vi "SwerveBegin.vi"() -> ()   [LabVIEW 2019]
uses:
  <vilib>/Rock Robotics/WPI/ThirdParty/Phoenix-LabVIEW/Motor Controller/Controls/CTRE_Phoenix_MotorControl_NeutralMode.ctl
panel:
  in  "PIDF":cluster{"P":dbl, "I":dbl, "D":dbl, "F":dbl}={"P"=0.1, "I"=0.0, "D"=0.0, "F"=0.0} {"P" format="%#_13g"}
  in  "Error In":errorcluster
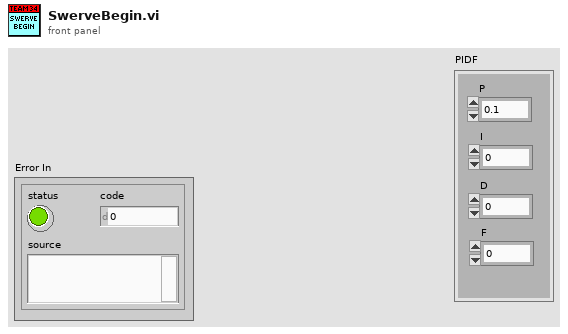
[diagram p1: front panel]
types:
  T1 = typedef "CTRE_Phoenix_MotorControl_NeutralMode.ctl" = enum8{"EEPROMSetting", "Override to Coast", "Override to Brake"}
  T2 = typedef "WPI_MotorControlDeviceRef.ctl" = cluster{"DeviceStatus":errorcluster, "Type":T3, "PWM":cluster{"PWM Channel":T4, "DeadBand":T5}, "CAN":cluster{"Device Number":u8, "SetOutput VI Ref":variant, "GetOutput VI Ref":variant, "Enable VI Ref":variant, "Disable VI Ref":variant, "Data":variant}, "Invert":bool, "DIO PWM":cluster{"PWM \"Enable\" Channel":T4, "DIOChannel":T6, "PWM Rate":dbl}}
  T3 = typedef "WPI_MotorControlType.ctl" = enum16{"PWM", "CAN", "DIO PWM"}
  T4 = typedef "FPGA_DIOPWMChannel.ctl" = enum8{"PWM 0", "PWM 1", "PWM 2", "PWM 3", "PWM 4", "PWM 5", "PWM 6", "PWM 7", "PWM 8", "PWM 9", "PWM MXP 0", "PWM MXP 1", "PWM MXP 2", "PWM MXP 3", "PWM MXP 4", "PWM MXP 5", "PWM MXP 6", "PWM MXP 7", "PWM MXP 8", "PWM MXP 9", "Invalid"}
  T5 = typedef "WPI_PWMDeadband.ctl" = cluster{"Name":string, "maxPositivePwm":i32, "minPositivePwm":i32, "centerPwm":i32, "maxNegativePwm":i32, "minNegativePwm":i32, "angularRange":u16}
  T6 = typedef "FPGA_DIOChannel.ctl" = enum8{"DIO 0", "DIO 1", "DIO 2", "DIO 3", "DIO 4", "DIO 5", "DIO 6", "DIO 7", "DIO 8", "DIO 9", "DIO MXP 0", "DIO MXP 1", "DIO MXP 2", "DIO MXP 3", "DIO MXP 4", "DIO MXP 5", "DIO MXP 6", "DIO MXP 7", "DIO MXP 8", "DIO MXP 9", "DIO MXP 10", "DIO MXP 11", "DIO MXP 12", "DIO MXP 13", "DIO MXP 14", "DIO MXP 15", "SPI Port CS1", "SPI Port CS2", "SPI Port CS3", "SPI Port MISO", "SPI Port MOSI", "Invalid"}
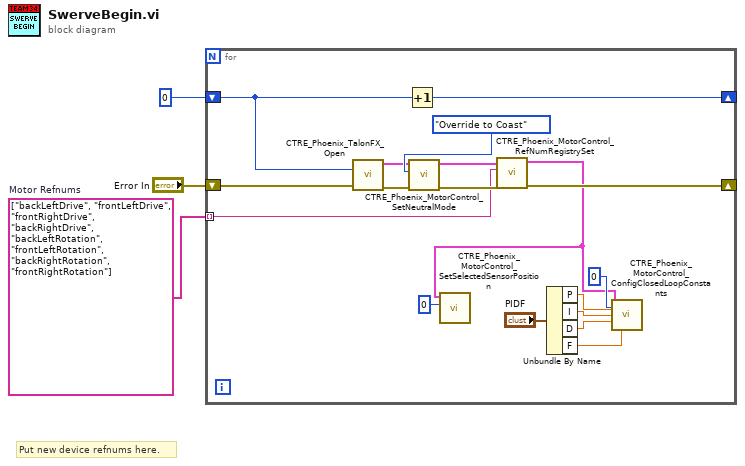
[diagram p0: block diagram]
diagram:
  w2 = string[] ["backLeftDrive", "frontLeftDrive", "frontRightDrive", "backRightDrive", "backLeftRotation", "frontLeftRotation", "backRightRotation", "frontRightRotation"]  # Motor Refnums
  # "Put new device refnums here."
  n1 = for {
    shift-right: [w21] -> _
    shift-left: u8 0 -> [w19]
    tunnel: w2 -> [w12] mode=indexing
    shift-right: [w13] -> _
    shift-left: "Error In" -> [w20]
    n2 = call <vilib>:"CTRE_Phoenix_TalonFX_Open.vi"("error in"=w20, "Device Number"=w19) -> ("error out"=w16:errorcluster, "CAN Talon SRX Ref"=w17:T2)  [unwired: 8 in]
    n3 = Increment(x=w19) -> (x+1=w21:u8)
    n4 = call <vilib>:"CTRE_Phoenix_MotorControl_SetNeutralMode.vi"("error in (no error)"=w16, "Motor Control Neutral Mode"=CTRE_Phoenix_MotorControl_NeutralMode."Override to Coast", "PhoenixMotorControlDevRef"=w17) -> ("error out"=w14:errorcluster, "PhoenixMotorControlDevRef"=w15:T2)  [unwired: 7 in]
    n5 = call <vilib>:"CTRE_Phoenix_MotorControl_RefNumRegistrySet.vi"("error in (no error)"=w14, "refnum name"=w12, "PhoenixMotorControlDevRef"=w15) -> ("error out"=w13:errorcluster, "PhoenixMotorControlDevRef"=w5:T2)  [unwired: 7 in]
    n6 = call <vilib>:"CTRE_Phoenix_MotorControl_SetSelectedSensorPosition.vi"("New Sensor Position"=0, "PhoenixMotorControlDevRef"=w5) -> ()  [unwired: 8 in, 2 out]
    n7 = Unbundle By Name("PIDF") -> ("P"=w6:dbl, "I"=w7:dbl, "D"=w8:dbl, "F"=w9:dbl)
    n8 = call <vilib>:"CTRE_Phoenix_MotorControl_ConfigClosedLoopConstants.vi"("PhoenixMotorControlDevRef"=w5, "slotIdx"=0, "P"=w6, "I"=w7, "D"=w8, "F"=w9) -> ()  [unwired: 8 in, 2 out]
  }
